vi "PQputCopyData.vi"(8 "error in (no error)":errorcluster, 9 "nbytes":i32, 10 "buffer":string) -> (0 "error out":errorcluster, 2 "PQputCopyData":i32)   [LabVIEW 2019, in "libpqlv64.lvlib"]
uses:
  libpqlv64.lvlib
  libpq.dll
panel:
  in  "conn":u32
  out "conn_out":u32
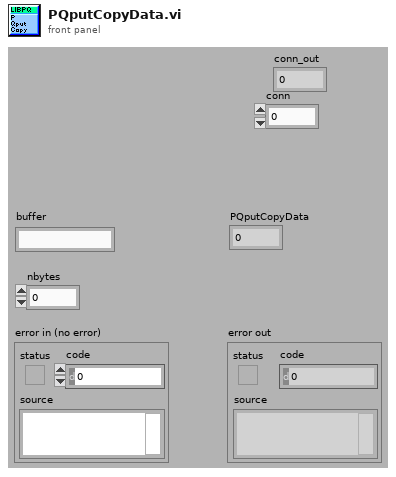
[diagram p1: front panel]
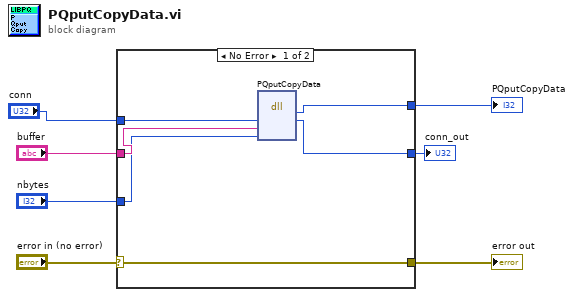
[diagram p0: block diagram]
diagram:
  n1 = case shown="No Error" "error in (no error)" {
    selector: "error in (no error)" -> [w13 w15]
    tunnel: [w13 w15] -> w6
    tunnel: [w12 _] -> w5
    tunnel: [w11 w14] -> w2
    tunnel: "buffer" -> [w10 _]
    tunnel: "nbytes" -> [w9 _]
    tunnel: "conn" -> [w8 w14]
    frame No Error {
      n2 = dll-call lib="libpq.*" fn="PQputCopyData"("conn"=w8, "buffer"=w10, "nbytes"=w9) -> ("PQputCopyData"=w12:i32, "conn"=w11:u32)  [unwired: 5 in, 2 out]
    }
    frame Error {
    }
  }
  "PQputCopyData" <- w5
  "error out" <- w6
  "conn_out" <- w2
